vi "Validate_Shortcuts.vi"(8 "error in (no error)":errorcluster, 11 "Installer in":refnum<class "Installer.lvclass">) -> (0 "error out":errorcluster, 3 "Installer out":refnum<class "Installer.lvclass">)   [LabVIEW 2020, in "Installer.lvclass"]
uses:
  <vilib>/AppBuilder/IB_Classes/Installer/Installer.lvclass
  <vilib>/AppBuilder/IB_Classes/Installer/Installer.lvclass/Installer.ctl
  <vilib>/AppBuilder/IB_Classes/Source/File/IB_Source_File.lvclass
  <vilib>/AppBuilder/IB_Classes/Source/IB_Source.lvclass
  <vilib>/AppBuilder/IB_Classes/Shortcut/IB_Shortcut.lvclass
  <resource>/Framework/Providers/Builds/Installer/CDK_sTypeDef_ShortcutAddress.ctl
  e:/builds/penguin/labview/branches/2020/dev/dist/vi.lib/AppBuilder/IB_Classes/Source/IB_Source.lvclass
  e:/builds/penguin/labview/branches/2020/dev/dist/vi.lib/AppBuilder/IB_Classes/Source/File/IB_Source_File.lvclass
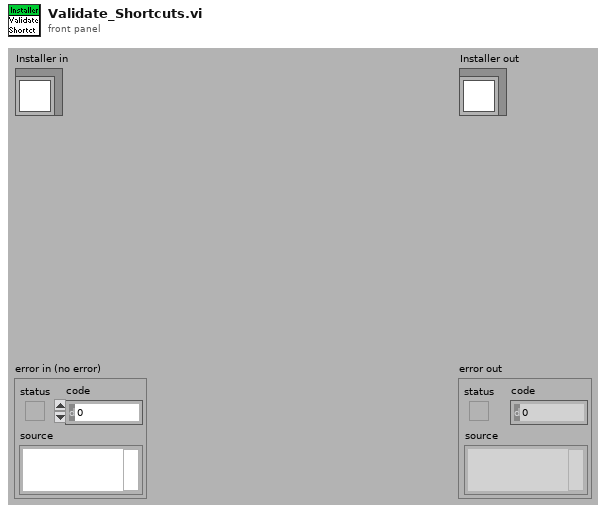
[diagram p1: front panel]
types:
  T1 = typedef "CDK_sTypeDef_ShortcutAddress.ctl" = cluster{"file":string, "shortcut":string}
  T2 = typedef "CDK_sTypeDef_FileList.ctl" = cluster{"FileInventory":refnum<class "IB_Source_File.lvclass">, "containerID":string}
  T3 = typedef "IB_Source_File.ctl" = cluster{"Attributes":i16, "RegCOM":bool, "unlock":bool, "shortcuts":refnum<class "IB_Shortcut.lvclass">[], "EXE_install":bool, "CmdArg_install":string, "EXE_uninstall":bool, "CmdArg_uninstall":string}
  T4 = typedef "IB_Source.ctl" = cluster{"name":string, "sourceTag":string, "destTag":string, "path":path, "eng_installPath":string, "UI_inBuild?":bool, "str ref?":bool}
  T5 = typedef "IB_Shortcut.ctl" = cluster{"name":string, "destIndex":i32, "subDir":string, "address":string}
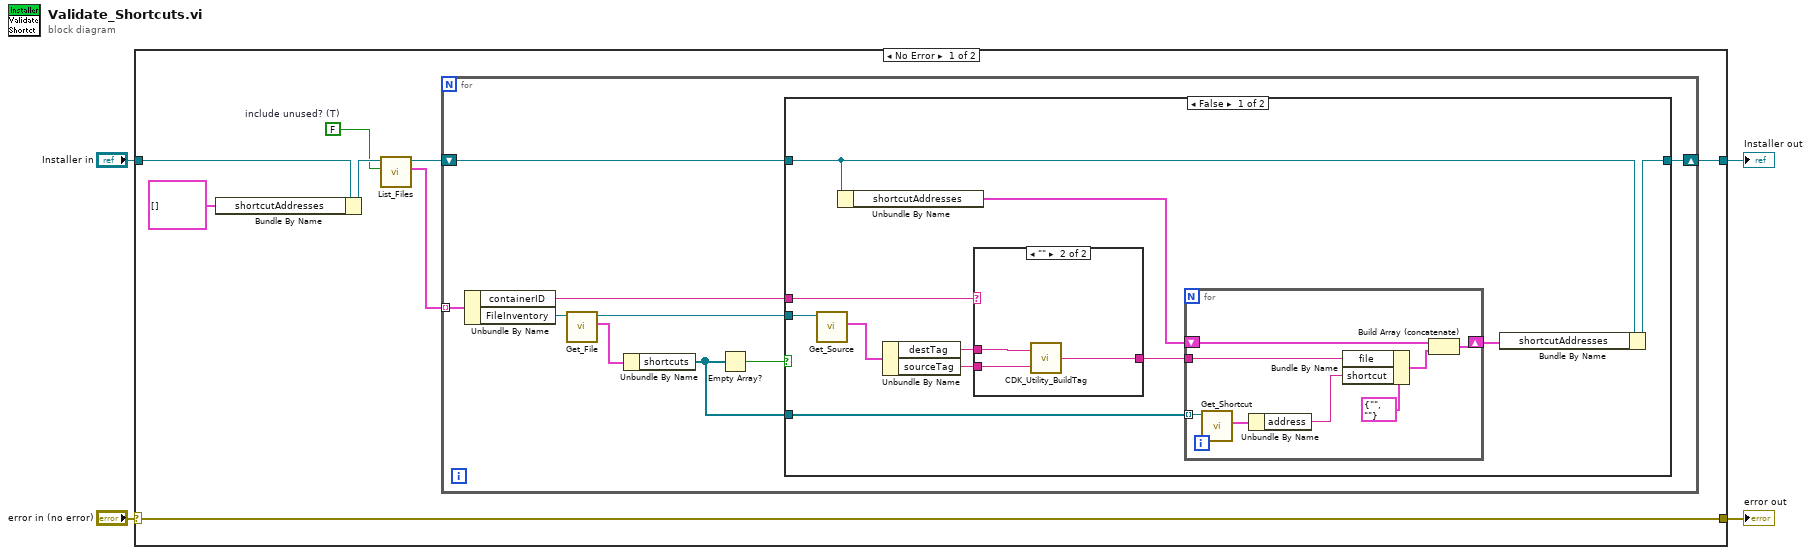
[diagram p0: block diagram]
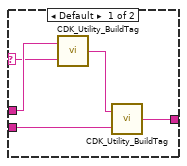
[diagram p2: hidden frame]
diagram:
  n1 = case shown="No Error" "error in (no error)" {
    selector: "error in (no error)" -> [w12 w51]
    tunnel: [w12 w51] -> w3
    tunnel: [w9 w50] -> w4
    tunnel: "Installer in" -> [w8 w50]
    frame No Error {
      w5 = FALSE  # include unused? (T)
      n2 = Bundle By Name(cluster=w8, "shortcutAddresses"=T1[] [] ("data.shortcutAddresses")) -> (w7:refnum<class "Installer.lvclass">)
      n3 = call <vilib>:"List_Files.vi"("include unused? (T)"=w5, "Installer in"=w7) -> ("files"=w11:T2[], "Installer out"=w10:refnum<class "Installer.lvclass">)  [unwired: 1 in, 7 out]
      n4 = for {
        tunnel: w11 -> [w20] mode=indexing
        shift-right: [w16] -> w9
        shift-left: w10 -> [w17]
        n5 = Unbundle By Name(w20) -> ("containerID"=w15:string, "FileInventory"=w19:refnum<class "IB_Source_File.lvclass">)
        n6 = call <vilib>:"Get_File.vi"("IB_Source_File in"=w19) -> ("data"=w21:T3, "IB_Source_File out"=w14:refnum<class "IB_Source_File.lvclass">)  [unwired: 1 in, 8 out]
        n7 = Unbundle By Name(w21) -> ("shortcuts"=w13:refnum<class "IB_Shortcut.lvclass">[])
        n8 = Empty Array?(array=w13) -> (empty?=w18:bool)
        n9 = case shown="False" w18 {
          tunnel: w14 -> [w31 _]
          tunnel: w15 -> [w28 _]
          tunnel: w17 -> [w26 w49]
          tunnel: [w27 w49] -> w16
          tunnel: w13 -> [w22 _]
          frame False {
            n10 = call <vilib>:"Get_Source.vi"("IB_Source in"=w31) -> ("data"=w32:T4)  [unwired: 1 in, 9 out]
            n11 = Unbundle By Name(w26) -> ("shortcutAddresses"=w25:T1[])
            n12 = Unbundle By Name(w32) -> ("destTag"=w30:string, "sourceTag"=w29:string)
            n13 = case shown="\"\"" w28 {
              selector: w28 -> [w44 _]
              tunnel: w30 -> [w45 w48]
              tunnel: w29 -> [w42 w47]
              tunnel: [w41 w46] -> w24
              frame Default {
                n14 = call <resource>:"CDK_Utility_BuildTag.vi"("name or relative path"=w44, "BasePath"=w45) -> ("appended path"=w43:string)
                n15 = call <resource>:"CDK_Utility_BuildTag.vi"("name or relative path"=w42, "BasePath"=w43) -> ("appended path"=w41:string)
              }
              frame "" {
                n16 = call <resource>:"CDK_Utility_BuildTag.vi"("name or relative path"=w47, "BasePath"=w48) -> ("appended path"=w46:string)
              }
            }
            n17 = for {
              tunnel: w24 -> [w35]
              tunnel: w22 -> [w38] mode=indexing
              shift-right: [w39] -> w23
              shift-left: w25 -> [w40]
              n18 = call <vilib>:"Get_Shortcut.vi"("Class in"=w38) -> ("data"=w37:T5)  [unwired: 1 in, 9 out]
              n19 = Unbundle By Name(w37) -> ("address"=w33:string)
              n20 = Bundle By Name(cluster=T1 {"file"="", "shortcut"=""} ("shortcut address"), "file"=w35, "shortcut"=w33) -> (w34:T1)
              n21 = Build Array (concatenate)(w40, w34) -> (w39:T1[])
            }
            n22 = Bundle By Name(cluster=w26, "shortcutAddresses"=w23) -> (w27:refnum<class "Installer.lvclass">)
          }
          frame True {
          }
        }
      }
    }
    frame Error {
    }
  }
  "error out" <- w3
  "Installer out" <- w4
